vi "Write_LS_Data_without_kelvinox.vi"(1 "In":T1={"Time"=[], "LI1CH1"=[], "LI1CH2"=[], "LI2CH1"=[], "LI2CH2"=[], "LI3CH1"=[], "LI3CH2"=[], "Field"=[], "N_Level"=[], "H_Level"=[], "Heat_370"=[], "Sorb_Heat"=[], "Still_Heat"=[], "Capacity"=[], "Loss"=[], "Magnet_Temperature"=[], "Lam_Pressure"=[], "Lam_NValve"=[], "370-T1"=[], "370-T2"=[], "370-T3"=[], "370-T4"=[], "370-T5"=[], "370-R1"=[], "370-R2"=[], "370-R3"=[], "370-R4"=[], "370-R5"=[], "372-T1"=[], "372-T2"=[], "372-T3"=[], "372-T4"=[], "372-T5"=[], "372-T6"=[], "372-R1"=[], "372-R2"=[], "372-R3"=[], "372-R4"=[], "372-R5"=[], "372-R6"=[], "Nada"=[nan], "K2440_Res"=[], "K2440_Current"=[], "VTI_Heater"=[], "VTI_NValve"=[], "LS340_Heater"=[], "K6221_Amplitude"=[], "K6221_Frequency"=[], "Cond_Pressure"=[], "Still_Pressure"=[], "FP_Out_Pressure"=[], "Dump_Pressure"=[], "V1"=[], "V2"=[], "V4"=[], "V5"=[], "V9"=[], "Forepump"=[], "Compressor"=[], "K6221_Offset"=[], "BoxTemp"=[], "By"=[], "Bz"=[], "Phi"=[], "heater-recond (%)"=[], "Dewar Pressure "=[], "JT-SP-Control"=[], "350 T1"=[], "350 T2"=[], "350 T3"=[], "350 T4"=[], "350 R1"=[], "350 R2"=[], "350 R3"=[], "350 R4"=[], "Angle"=[], "VTI CH1"=[], "VTI CH2"=[], "VTI CH3"=[], "ColdTrap"=[], "Mischer Pot"=[], "G1 (mbar)"=[], "G3 (mbar) "=[], "G4 (mbar)"=[], "IVC (mbar)"=[], "P2 (mbar) "=[], "Pot mischer (mbar)"=[], "AVS Control Channel (K)"=[], "AVS Control Channel (RES)"=[], "AVS  Channel 5 (RES) "=[], "LI3CH3"=[], "LI3CH4"=[], "LI1CH3"=[], "LI1CH4"=[], "LI2CH3"=[], "LI2CH4"=[], "Volt"=[], "Watt"=[], "Torque Angle"=[], "Dewar heater (W)"=[], "PSU Voltage"=[], "Turbopump"=[], "372-R7"=[], "372-T7"=[], "SIM921 Ch1"=[], " He3 Temp1"=[], " He3 Temp 2"=[], "LI4CH1"=[], "LI4CH2"=[], "372-T8"=[], "372-R8"=[]}) -> (0 "Out":T1={"Time"=[], "LI1CH1"=[], "LI1CH2"=[], "LI2CH1"=[], "LI2CH2"=[], "LI3CH1"=[], "LI3CH2"=[], "Field"=[], "N_Level"=[], "H_Level"=[], "Heat_370"=[], "Sorb_Heat"=[], "Still_Heat"=[], "Capacity"=[], "Loss"=[], "Magnet_Temperature"=[], "Lam_Pressure"=[], "Lam_NValve"=[], "370-T1"=[], "370-T2"=[], "370-T3"=[], "370-T4"=[], "370-T5"=[], "370-R1"=[], "370-R2"=[], "370-R3"=[], "370-R4"=[], "370-R5"=[], "372-T1"=[], "372-T2"=[], "372-T3"=[], "372-T4"=[], "372-T5"=[], "372-T6"=[], "372-R1"=[], "372-R2"=[], "372-R3"=[], "372-R4"=[], "372-R5"=[], "372-R6"=[], "Nada"=[nan], "K2440_Res"=[], "K2440_Current"=[], "VTI_Heater"=[], "VTI_NValve"=[], "LS340_Heater"=[], "K6221_Amplitude"=[], "K6221_Frequency"=[], "Cond_Pressure"=[], "Still_Pressure"=[], "FP_Out_Pressure"=[], "Dump_Pressure"=[], "V1"=[], "V2"=[], "V4"=[], "V5"=[], "V9"=[], "Forepump"=[], "Compressor"=[], "K6221_Offset"=[], "BoxTemp"=[], "By"=[], "Bz"=[], "Phi"=[], "heater-recond (%)"=[], "Dewar Pressure "=[], "JT-SP-Control"=[], "350 T1"=[], "350 T2"=[], "350 T3"=[], "350 T4"=[], "350 R1"=[], "350 R2"=[], "350 R3"=[], "350 R4"=[], "Angle"=[], "VTI CH1"=[], "VTI CH2"=[], "VTI CH3"=[], "ColdTrap"=[], "Mischer Pot"=[], "G1 (mbar)"=[], "G3 (mbar) "=[], "G4 (mbar)"=[], "IVC (mbar)"=[], "P2 (mbar) "=[], "Pot mischer (mbar)"=[], "AVS Control Channel (K)"=[], "AVS Control Channel (RES)"=[], "AVS  Channel 5 (RES) "=[], "LI3CH3"=[], "LI3CH4"=[], "LI1CH3"=[], "LI1CH4"=[], "LI2CH3"=[], "LI2CH4"=[], "Volt"=[], "Watt"=[], "Torque Angle"=[], "Dewar heater (W)"=[], "PSU Voltage"=[], "Turbopump"=[], "372-R7"=[], "372-T7"=[], "SIM921 Ch1"=[], " He3 Temp1"=[], " He3 Temp 2"=[], "LI4CH1"=[], "LI4CH2"=[], "372-T8"=[], "372-R8"=[]})   [LabVIEW 2019]
uses:
  Global/Global Variables/System Monitor Cluster.ctl
  Global/Global Variables/Data_Display_global.vi
  Instrument_Setup.vi
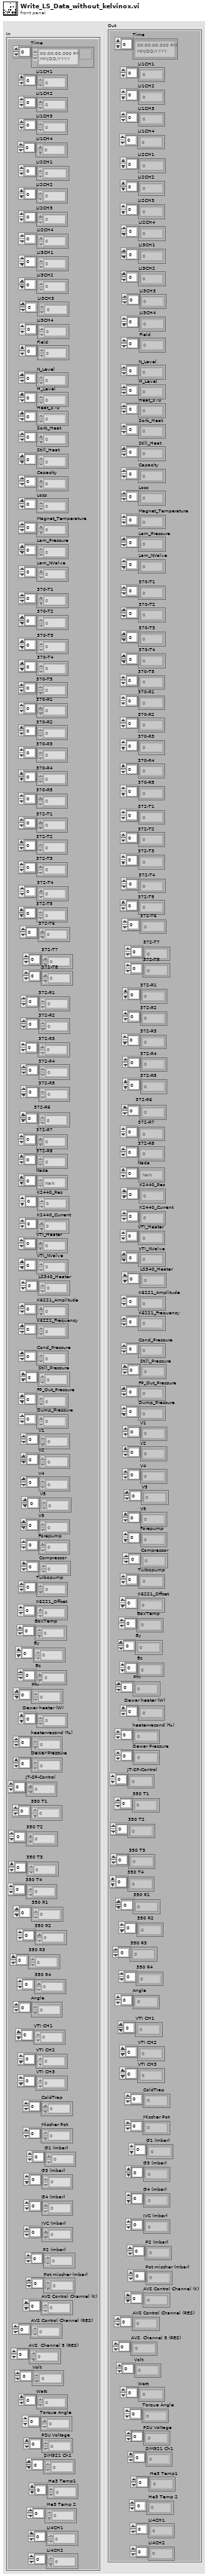
[diagram p1: front panel]
types:
  T1 = typedef "System Monitor Cluster.ctl" = cluster{"Time":timestamp[], "LI1CH1":dbl[], "LI1CH2":dbl[], "LI2CH1":dbl[], "LI2CH2":dbl[], "LI3CH1":dbl[], "LI3CH2":dbl[], "Field":dbl[], "N_Level":dbl[], "H_Level":dbl[], "Heat_370":dbl[], "Sorb_Heat":dbl[], "Still_Heat":dbl[], "Capacity":dbl[], "Loss":dbl[], "Magnet_Temperature":dbl[], "Lam_Pressure":dbl[], "Lam_NValve":dbl[], "370-T1":dbl[], "370-T2":dbl[], "370-T3":dbl[], "370-T4":dbl[], "370-T5":dbl[], "370-R1":dbl[], "370-R2":dbl[], "370-R3":dbl[], "370-R4":dbl[], "370-R5":dbl[], "372-T1":dbl[], "372-T2":dbl[], "372-T3":dbl[], "372-T4":dbl[], "372-T5":dbl[], "372-T6":dbl[], "372-R1":dbl[], "372-R2":dbl[], "372-R3":dbl[], "372-R4":dbl[], "372-R5":dbl[], "372-R6":dbl[], "Nada":dbl[], "K2440_Res":dbl[], "K2440_Current":dbl[], "VTI_Heater":dbl[], "VTI_NValve":dbl[], "LS340_Heater":dbl[], "K6221_Amplitude":dbl[], "K6221_Frequency":dbl[], "Cond_Pressure":dbl[], "Still_Pressure":dbl[], "FP_Out_Pressure":dbl[], "Dump_Pressure":dbl[], "V1":dbl[], "V2":dbl[], "V4":dbl[], "V5":dbl[], "V9":dbl[], "Forepump":dbl[], "Compressor":dbl[], "K6221_Offset":dbl[], "BoxTemp":dbl[], "By":dbl[], "Bz":dbl[], "Phi":dbl[], "heater-recond (%)":dbl[], "Dewar Pressure ":dbl[], "JT-SP-Control":dbl[], "350 T1":dbl[], "350 T2":dbl[], "350 T3":dbl[], "350 T4":dbl[], "350 R1":dbl[], "350 R2":dbl[], "350 R3":dbl[], "350 R4":dbl[], "Angle":dbl[], "VTI CH1":dbl[], "VTI CH2":dbl[], "VTI CH3":dbl[], "ColdTrap":dbl[], "Mischer Pot":dbl[], "G1 (mbar)":dbl[], "G3 (mbar) ":dbl[], "G4 (mbar)":dbl[], "IVC (mbar)":dbl[], "P2 (mbar) ":dbl[], "Pot mischer (mbar)":dbl[], "AVS Control Channel (K)":dbl[], "AVS Control Channel (RES)":dbl[], "AVS  Channel 5 (RES) ":dbl[], "LI3CH3":dbl[], "LI3CH4":dbl[], "LI1CH3":dbl[], "LI1CH4":dbl[], "LI2CH3":dbl[], "LI2CH4":dbl[], "Volt":dbl[], "Watt":dbl[], "Torque Angle":dbl[], "Dewar heater (W)":dbl[], "PSU Voltage":dbl[], "Turbopump":dbl[], "372-R7":dbl[], "372-T7":dbl[], "SIM921 Ch1":dbl[], " He3 Temp1":dbl[], " He3 Temp 2":dbl[], "LI4CH1":dbl[], "LI4CH2":dbl[], "372-T8":dbl[], "372-R8":dbl[]}
  T2 = typedef "LS370_only_readout_cluster.ctl" = cluster{"LS370 T1":dbl, "LS370 T2":dbl, "LS370 T3":dbl, "LS370 T4":dbl, "LS370 T5":dbl, "LS370 R1":dbl, "LS370 R2":dbl, "LS370 R3":dbl, "LS370 R4":dbl, "LS370 R5":dbl, "LS370 T6":dbl, "LS370 T7":dbl, "LS370 T8":dbl, "LS370 T9":dbl, "LS370 R6":dbl, "LS370 R7":dbl, "LS370 R8":dbl, "LS370 R9":dbl, "LS370 TC-T":dbl, "LS370 TC-R":dbl, "Update Lakeshores":bool}
  T3 = typedef "LS370_Status.ctl" = cluster{"Setpoint":dbl, "MC Heater Output":dbl, "Still Heater Output":dbl, "Sorb  Heater Output":dbl, "LS370 T1":dbl, "LS370 T2":dbl, "LS370 T3":dbl, "LS370 T4":dbl, "LS370 T5":dbl, "LS370 R1":dbl, "LS370 R2":dbl, "LS370 R3":dbl, "LS370 R4":dbl, "LS370 R5":dbl, "LS370 T6":dbl, "LS370 T7":dbl, "LS370 T8":dbl, "LS370 T9":dbl, "LS370 R6":dbl, "LS370 R7":dbl, "LS370 R8":dbl, "LS370 R9":dbl, "LS370 TC-T":dbl, "LS370 TC-R":dbl}
  T4 = typedef "LS350-cluster.ctl" = cluster{"Setpoint":dbl, "Heater Output":dbl, "Setpoint control":dbl, "Enable Setpoint":bool, "LS350 T1":dbl, "LS350 T2":dbl, "LS350 T3":dbl, "LS350 T4":dbl, "LS350 R1":dbl, "LS350 R2":dbl, "LS350 R3":dbl, "LS350 R4":dbl}
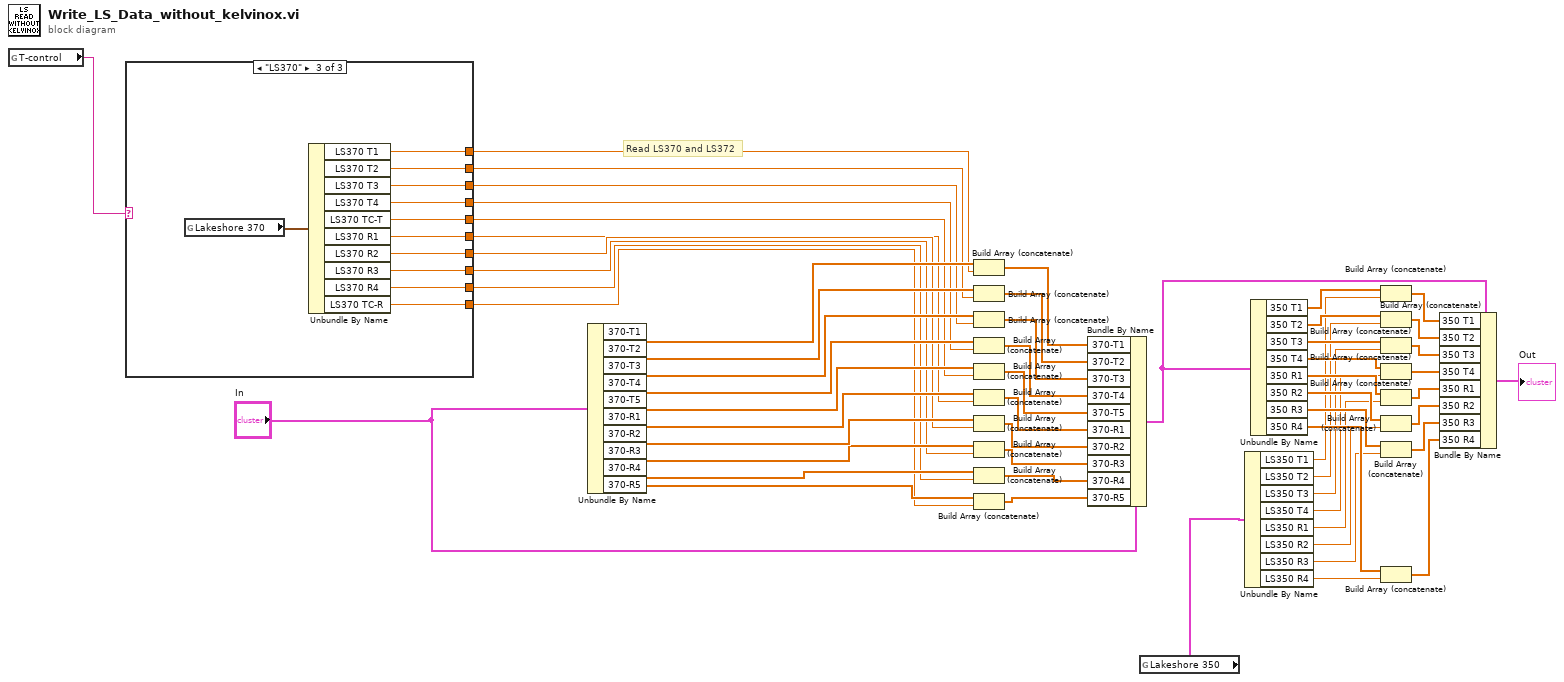
[diagram p0: block diagram]
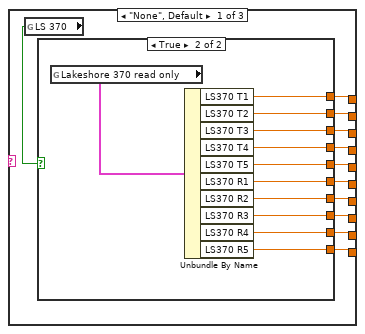
[diagram p2: hidden frame]
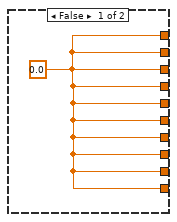
[diagram p3: hidden frame]
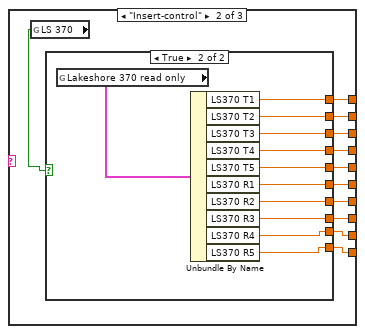
[diagram p4: hidden frame]
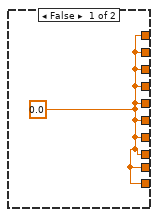
[diagram p5: hidden frame]
diagram:
  # "Read LS370 and LS372"
  n1 = global read "Instrument_Setup.vi" "T-control"() -> (w1:string)
  n2 = case shown="\"LS370\"" w1 {
    tunnel: [w68 w91 w114] -> w38
    tunnel: [w69 w92 w115] -> w37
    tunnel: [w67 w90 w113] -> w36
    tunnel: [w66 w89 w112] -> w35
    tunnel: [w63 w86 w109] -> w34
    tunnel: [w62 w85 w108] -> w33
    tunnel: [w61 w84 w107] -> w32
    tunnel: [w60 w83 w106] -> w31
    tunnel: [w65 w88 w111] -> w30
    tunnel: [w64 w87 w110] -> w29
    frame "None", Default {
      n3 = global read "Instrument_Setup.vi" "LS 370"() -> (w70:bool)
      n4 = case shown="True" w70 {
        tunnel: [w71 w81] -> w69
        tunnel: [w71 w80] -> w68
        tunnel: [w71 w79] -> w67
        tunnel: [w71 w78] -> w66
        tunnel: [w71 w77] -> w65
        tunnel: [w71 w76] -> w64
        tunnel: [w71 w75] -> w63
        tunnel: [w71 w74] -> w62
        tunnel: [w71 w73] -> w61
        tunnel: [w71 w72] -> w60
        frame False {
          w71 = 0.0
        }
        frame True {
          n5 = global read "Data_Display_global.vi" "Lakeshore 370 read only"() -> (w82:T2)
          n6 = Unbundle By Name(w82) -> ("LS370 T1"=w81:dbl, "LS370 T2"=w80:dbl, "LS370 T3"=w79:dbl, "LS370 T4"=w78:dbl, "LS370 T5"=w77:dbl, "LS370 R1"=w76:dbl, "LS370 R2"=w75:dbl, "LS370 R3"=w74:dbl, "LS370 R4"=w73:dbl, "LS370 R5"=w72:dbl)
        }
      }
    }
    frame "Insert-control" {
      n7 = global read "Instrument_Setup.vi" "LS 370"() -> (w93:bool)
      n8 = case shown="True" w93 {
        tunnel: [w94 w104] -> w92
        tunnel: [w94 w103] -> w91
        tunnel: [w94 w102] -> w90
        tunnel: [w94 w101] -> w89
        tunnel: [w94 w100] -> w88
        tunnel: [w94 w99] -> w87
        tunnel: [w94 w98] -> w86
        tunnel: [w94 w97] -> w85
        tunnel: [w94 w96] -> w84
        tunnel: [w94 w95] -> w83
        frame False {
          w94 = 0.0
        }
        frame True {
          n9 = global read "Data_Display_global.vi" "Lakeshore 370 read only"() -> (w105:T2)
          n10 = Unbundle By Name(w105) -> ("LS370 T1"=w104:dbl, "LS370 T2"=w103:dbl, "LS370 T3"=w102:dbl, "LS370 T4"=w101:dbl, "LS370 T5"=w100:dbl, "LS370 R1"=w99:dbl, "LS370 R2"=w98:dbl, "LS370 R3"=w97:dbl, "LS370 R4"=w96:dbl, "LS370 R5"=w95:dbl)
        }
      }
    }
    frame "LS370" {
      n11 = global read "Data_Display_global.vi" "Lakeshore 370"() -> (w116:T3)
      n12 = Unbundle By Name(w116) -> ("LS370 T1"=w115:dbl, "LS370 T2"=w114:dbl, "LS370 T3"=w113:dbl, "LS370 T4"=w112:dbl, "LS370 TC-T"=w111:dbl, "LS370 R1"=w110:dbl, "LS370 R2"=w109:dbl, "LS370 R3"=w108:dbl, "LS370 R4"=w107:dbl, "LS370 TC-R"=w106:dbl)
    }
  }
  n13 = Unbundle By Name("In") -> ("370-T1"=w59:dbl[], "370-T2"=w58:dbl[], "370-T3"=w57:dbl[], "370-T4"=w56:dbl[], "370-T5"=w55:dbl[], "370-R1"=w54:dbl[], "370-R2"=w53:dbl[], "370-R3"=w52:dbl[], "370-R4"=w51:dbl[], "370-R5"=w50:dbl[])
  n14 = Build Array (concatenate)(w59, w37) -> (w49:dbl[])
  n15 = Build Array (concatenate)(w58, w38) -> (w48:dbl[])
  n16 = Build Array (concatenate)(w57, w36) -> (w47:dbl[])
  n17 = Build Array (concatenate)(w56, w35) -> (w46:dbl[])
  n18 = Build Array (concatenate)(w55, w30) -> (w45:dbl[])
  n19 = Build Array (concatenate)(w54, w29) -> (w44:dbl[])
  n20 = Build Array (concatenate)(w53, w34) -> (w43:dbl[])
  n21 = Build Array (concatenate)(w52, w33) -> (w42:dbl[])
  n22 = Build Array (concatenate)(w51, w32) -> (w41:dbl[])
  n23 = Build Array (concatenate)(w50, w31) -> (w40:dbl[])
  n24 = Bundle By Name(cluster="In", "370-T1"=w49, "370-T2"=w48, "370-T3"=w47, "370-T4"=w46, "370-T5"=w45, "370-R1"=w44, "370-R2"=w43, "370-R3"=w42, "370-R4"=w41, "370-R5"=w40) -> (w11:T1)
  n25 = global read "Data_Display_global.vi" "Lakeshore 350"() -> (w28:T4)
  n26 = Unbundle By Name(w28) -> ("LS350 T1"=w12:dbl, "LS350 T2"=w13:dbl, "LS350 T3"=w14:dbl, "LS350 T4"=w15:dbl, "LS350 R1"=w16:dbl, "LS350 R2"=w17:dbl, "LS350 R3"=w18:dbl, "LS350 R4"=w19:dbl)
  n27 = Unbundle By Name(w11) -> ("350 T1"=w27:dbl[], "350 T2"=w26:dbl[], "350 T3"=w25:dbl[], "350 T4"=w24:dbl[], "350 R1"=w23:dbl[], "350 R2"=w22:dbl[], "350 R3"=w21:dbl[], "350 R4"=w20:dbl[])
  n28 = Build Array (concatenate)(w27, w12) -> (w9:dbl[])
  n29 = Build Array (concatenate)(w26, w13) -> (w8:dbl[])
  n30 = Build Array (concatenate)(w25, w14) -> (w7:dbl[])
  n31 = Build Array (concatenate)(w24, w15) -> (w6:dbl[])
  n32 = Build Array (concatenate)(w23, w16) -> (w5:dbl[])
  n33 = Build Array (concatenate)(w22, w17) -> (w4:dbl[])
  n34 = Build Array (concatenate)(w21, w18) -> (w3:dbl[])
  n35 = Build Array (concatenate)(w20, w19) -> (w2:dbl[])
  n36 = Bundle By Name(cluster=w11, "350 T1"=w9, "350 T2"=w8, "350 T3"=w7, "350 T4"=w6, "350 R1"=w5, "350 R2"=w4, "350 R3"=w3, "350 R4"=w2) -> (→"Out":T1)
